vi "Setup.vi"(0 "SG Path Group in":refnum<class "SG 18GHz Path Group.lvclass">, 11 "error in (no error)":errorcluster) -> (4 "SG Path Group out":refnum<class "SG 18GHz Path Group.lvclass">, 15 "error out":errorcluster)   [LabVIEW 2023, in "RFFixtureCharact.RFPM.lvlib" / "SG 18GHz Path Group.lvclass"]
uses:
  SG 18GHz Path Group.lvclass
  Public/Base Classes/Scalar/Scalar Path Group/Scalar Path Group.lvclass
  Instruments/Power Meter/Power Meter Base/Power Meter Base.lvclass
  Common/RFCalAndFixtureCharact.Common.lvlib
  Instruments/Power Meter/Power Meter Factory/Power Meter Factory.lvclass
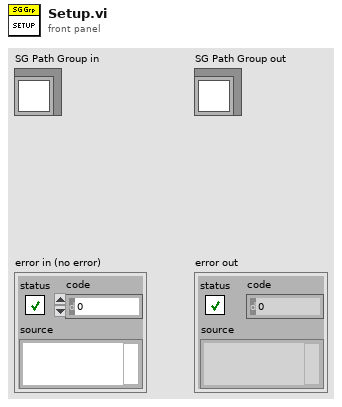
[diagram p1: front panel]
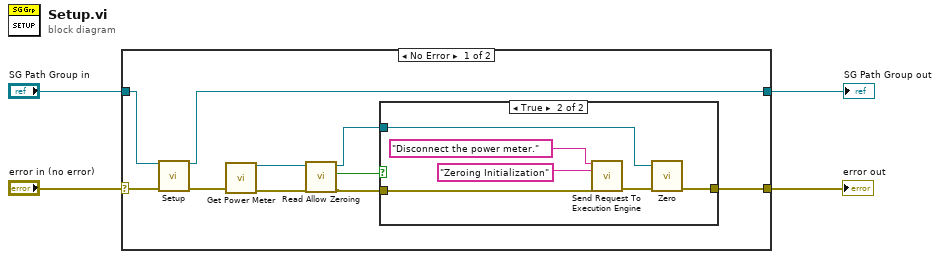
[diagram p0: block diagram]
diagram:
  n1 = case shown="No Error" "error in (no error)" {
    selector: "error in (no error)" -> [w14 w22]
    tunnel: [w5 w22] -> w4
    tunnel: "SG Path Group in" -> [w13 w23]
    tunnel: [w12 w23] -> w1
    frame No Error {
      n2 = call-parent "Setup.vi"("Path Group in"=w13, "error in"=w14) -> ("Path Group out"=w12:refnum<class "SG 18GHz Path Group.lvclass">, "error out"=w11:errorcluster)  [unwired: 12 in]
      n3 = call "Get Power Meter.vi"("error in (no error)"=w11) -> ("Power Meter Base out"=w10:refnum<class "Power Meter Base.lvclass">, "error out"=w9:errorcluster)  [unwired: 13 in]
      n4 = call-dynamic "Read Allow Zeroing.vi"("error in (no error)"=w9, "Power Meter Base in"=w10) -> ("error out"=w8:errorcluster, "Allow Zeroing"=w7:bool, "Power Meter Base out"=w6:refnum<class "Power Meter Base.lvclass">)  [unwired: 7 in]
      n5 = case shown="True" w7 {
        tunnel: w8 -> [w15 w19]
        tunnel: w6 -> [_ w18]
        tunnel: [w15 w16] -> w5
        frame False {
        }
        frame True {
          n6 = call "Send Request To Execution Engine.vi"("Request Message"="Disconnect the power meter." ("message"), "Request Header"="Zeroing Initialization", "error in (no error)"=w19) -> ("error out"=w17:errorcluster)  [unwired: 11 in, 1 out]
          n7 = call-dynamic "Zero.vi"("Power Meter Base in"=w18, "error in (no error)"=w17) -> ("error out"=w16:errorcluster)  [unwired: 12 in, 1 out]
        }
      }
    }
    frame Error {
    }
  }
  "error out" <- w4
  "SG Path Group out" <- w1
